vi "SingleValuetoArrayofSix.vi"(8 "error in (no error)":errorcluster, 10 "Numeric":dbl, 11 "Connected Axes":string[](array[string])) -> (0 "error out":errorcluster, 2 "Array":dbl[](array[numeric]))   [LabVIEW 2020]
doc: "This takes in one number and makes a 1D array with 6 of that number"
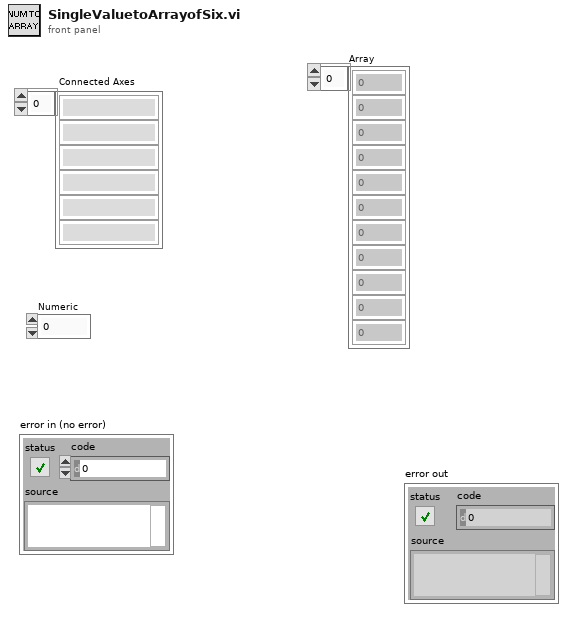
[diagram p1: front panel]
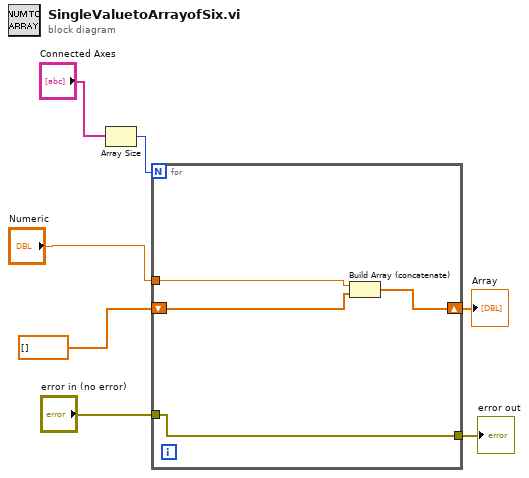
[diagram p0: block diagram]
diagram:
  n1 = Array Size(array="Connected Axes") -> (size(s)=w1:i32)
  n2 = for {
    N: w1 -> [_]
    tunnel: "Numeric" -> [w11]
    shift-right: [w10] -> w6
    shift-left: dbl[] [] -> [w9]
    tunnel: "error in (no error)" -> [w8]
    tunnel: [w8] -> w3
    n3 = Build Array (concatenate)(w11, w9) -> (w10:dbl[])
  }
  "Array" <- w6
  "error out" <- w3
